vi "Get End Tag.vi"(8 "error in (no error)":errorcluster, 10 "Name":string, 11 "Attribute in":refnum<class "Attribute.lvclass">) -> (0 "error out":errorcluster, 2 "End Tag":string, 3 "Attribute out":refnum<class "Attribute.lvclass">)   [LabVIEW 2026, in "VILab.lvlib" / "Attribute.lvclass"]
uses:
  Attribute.lvclass
  Data Item/Data Item.lvclass
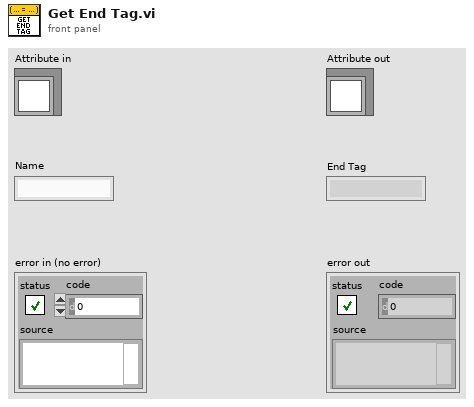
[diagram p1: front panel]
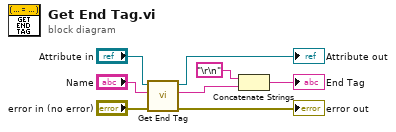
[diagram p0: block diagram]
diagram:
  n1 = call-parent "Get End Tag.vi"("error in (no error)"="error in (no error)", "Name"="Name", "Data Item in"="Attribute in") -> ("error out"=→"error out":errorcluster, "End Tag"=w2:string, "Data Item out"=→"Attribute out":refnum<class "Attribute.lvclass">)  [unwired: 6 in]
  n2 = Concatenate Strings("\r\n", w2) -> (→"End Tag":string)
